vi "Letters to Value Lookup.vi"() -> (3 "map in":map{string, i32}(c390))   [LabVIEW 2021]
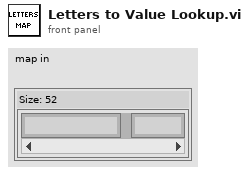
[diagram p1: front panel]
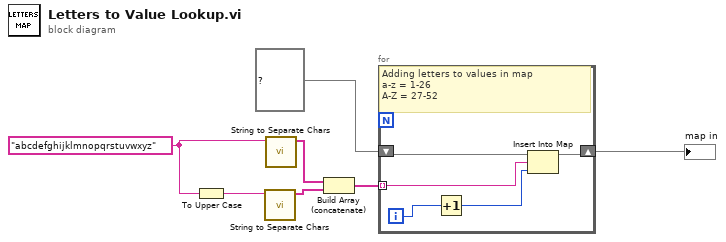
[diagram p0: block diagram]
diagram:
  w7 = "abcdefghijklmnopqrstuvwxyz"
  n1 = To Upper Case(1:w7) -> (0:w6:string)
  n2 = call "String to Separate Chars.vi"("String"=w6) -> ("Array"=w4:string[])  [unwired: 10 in]
  n3 = call "String to Separate Chars.vi"("String"=w7) -> ("Array"=w5:string[])  [unwired: 10 in]
  n4 = Build Array (concatenate)(w5, w4) -> (w2:string[])
  n5 = for {
    tunnel: w2 -> [w9] mode=indexing
    shift-right: [w8] -> w1
    shift-left: map{string, i32} {} ("map in") -> [w12]
    i -> [w11]
    # "Adding letters to values in map\na-z = 1-26\nA-Z = 27-52"
    n6 = Increment(x=w11) -> (x+1=w10:i32)
    n7 = Insert Into Map(map in=w12, key=w9, value=w10) -> (map out=w8:map{string, i32})  [unwired: 2 out]
  }
  "map in" <- w1
